vi "Write Reports.vi"(8 "error in (no error)":errorcluster, 10 "Reports":refnum<class "Report Data.lvclass">[](array[class]), 11 "Report Action in":refnum<class "Report Action.lvclass">) -> (0 "error out":errorcluster, 3 "Report Action out":refnum<class "Report Action.lvclass">)   [LabVIEW 2020]
uses:
  Report Action.lvclass
  Data/Report Data/Report Data.lvclass
  Report Action.lvclass/Report Action.ctl
  C:/Current projects/WS/LV32.2020..ProjectBuilder/Class/Action/Project Action/Project Action.lvclass
  C:/Current projects/WS/LV32.2020..ProjectBuilder/Interface/Action Interface/Action Interface.lvclass
  C:/Current projects/WS/LV32.2020..ProjectBuilder/Class/Report Action/Report Action/Report Action.lvclass
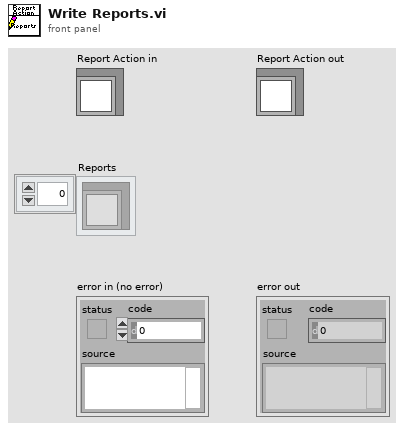
[diagram p1: front panel]
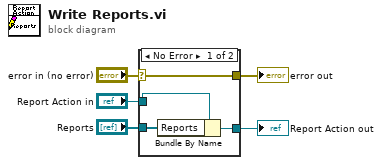
[diagram p0: block diagram]
diagram:
  n1 = case shown="No Error" "error in (no error)" {
    selector: "error in (no error)" -> [w9 w10]
    tunnel: [w9 w10] -> w4
    tunnel: [w7 w11] -> w2
    tunnel: "Report Action in" -> [w8 w11]
    tunnel: "Reports" -> [w6 _]
    frame No Error {
      n2 = Bundle By Name(cluster=w8, "Reports"=w6) -> (w7:refnum<class "Report Action.lvclass">)
    }
    frame Error {
    }
  }
  "error out" <- w4
  "Report Action out" <- w2
